vi "Fitter.vi"(8 "error in (no error)":errorcluster, 11 "PmuAnalysis in":refnum<class "FreqAnalysis.lvclass">) -> (0 "error out":errorcluster, 3 "PmuAnalysis out":refnum<class "FreqAnalysis.lvclass">)   [LabVIEW 2018, in "AnalysisPlugins.lvlib" / "FreqAnalysis.lvclass"]
uses:
  FreqAnalysis.lvclass
  C:/projects/ICDAS/NistPluggableModules/Analysis/AnalysisPlugins/AnalysisPluginBaseClass/AnalysisPluginsBase.lvclass
  C:/projects/ICDAS/NistPluggableModules/Analysis/AnalysisPlugins/PmuAnalysisClass/PmuAnalysis.lvclass
  AnalysisPluginBaseClass/AnalysisPluginsBase.lvclass/AnalysisPluginsBase.ctl
  PmuAnalysisClass/Typedefs/PmuData.ctl
  <vilib>/Analysis/coordinate.llb/Angle Units.ctl
  <vilib>/Analysis/coordinate.llb/Angle Range (Degree).ctl
  FitterBaseClass/Typedefs/clAnalysisConfig.ctl
  PmuAnalysisClass/PmuAnalysis.lvclass/PmuAnalysis.ctl
  <vilib>/Analysis/coordinate.llb/Wrap Angle (scalar).vi
  PmuAnalysisClass/Accessors/Read eTestType.vi
  AnalysisPluginBaseClass/Accessors/Read DelayCorr.vi
  AnalysisPluginBaseClass/Accessors/Read MagCorr.vi
  AnalysisPluginBaseClass/Accessors/Read AnalysisConfig.vi
  PmuAnalysisClass/Accessors/Read Function.vi
  PmuAnalysisClass/Accessors/Write Reference.vi
  AnalysisPluginBaseClass/Accessors/Read Window.vi
  <vilib>/Utility/error.llb/Error Cluster From Error Code.vi
  FGen/MemberClasses/FunctionBaseClass/FunctionBase.lvclass
  <vilib>/ErrorRing/Error Ring.xnode
  <vilib>/Analysis/NI_AAL_Angle.lvlib
  PmuAnalysisClass/PmuAnalysis.lvclass
  FitterBaseClass/FitterBase.lvclass
panel:
  out "Phase (rad)":dbl[](array[numeric])
  out "Magnitude":dbl[](array[numeric])
  out "Waveform Graph":dbl[][](graph)
  out "iterations":i32[](array[numeric])
  out "theta":dbl
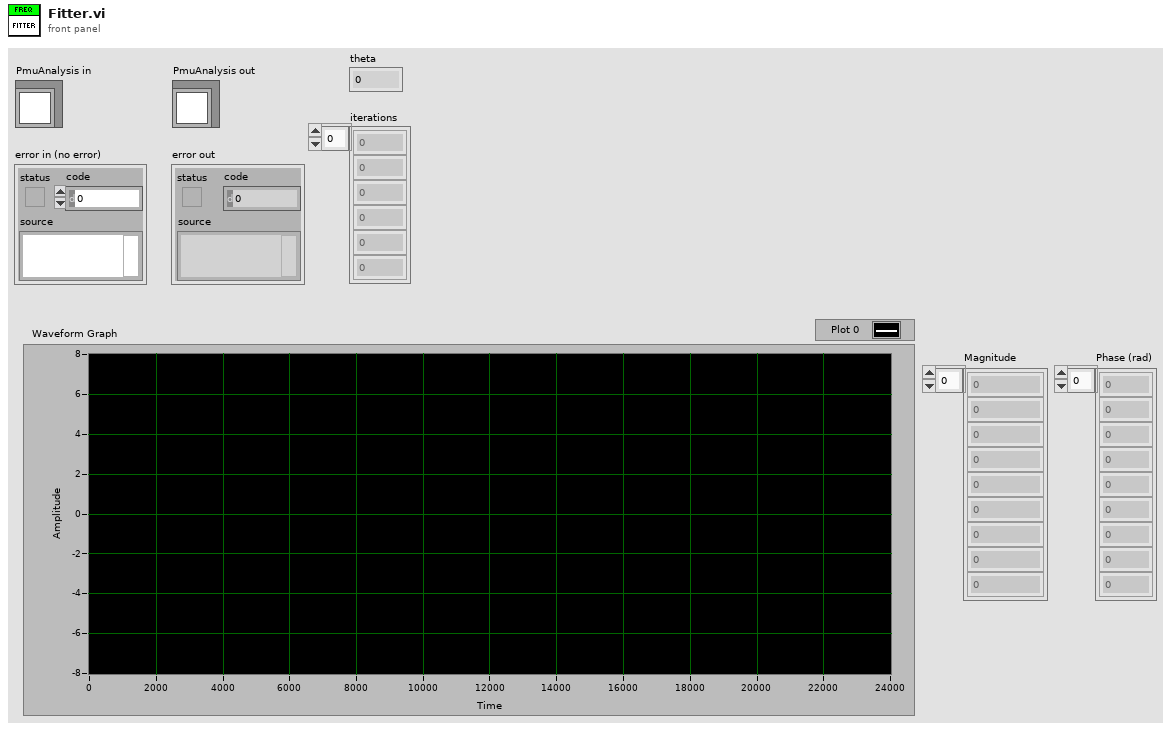
[diagram p1: front panel]
types:
  T1 = typedef "AnalysisPlugins.lvlib/FitterBase.lvclass/clAnalysisConfig.ctl" = cluster{"F0":u32, "SettlingTime":dbl, "AnalysisCycles":dbl, "SampleRate":dbl, "NumChannels":u32, "TsOffset":enum16{"start", "middle", "end"}}
  T2 = typedef "AnalysisPlugins.lvlib/PmuAnalysis.lvclass/PmuData.ctl" = cluster{"Timestamp":dbl, "Synx":cdb[], "Freq":dbl, "ROCOF":dbl, "ID":i16}
  T3 = typedef "AnalysisPlugins.lvlib/AnalysisPluginsBase.lvclass/clWindowData.ctl" = cluster{"Timestamp":ext, "Samples":dbl[][], "Window Valid":bool, "T0":ext}
  T4 = typedef "NI_AAL_Angle.lvlib/Angle Range (Degree).ctl" = u16
  T5 = typedef "NI_AAL_Angle.lvlib/Angle Units.ctl" = i32
  T6 = enum16{"SteadyState", "Modulation", "Ramp", "Step"}
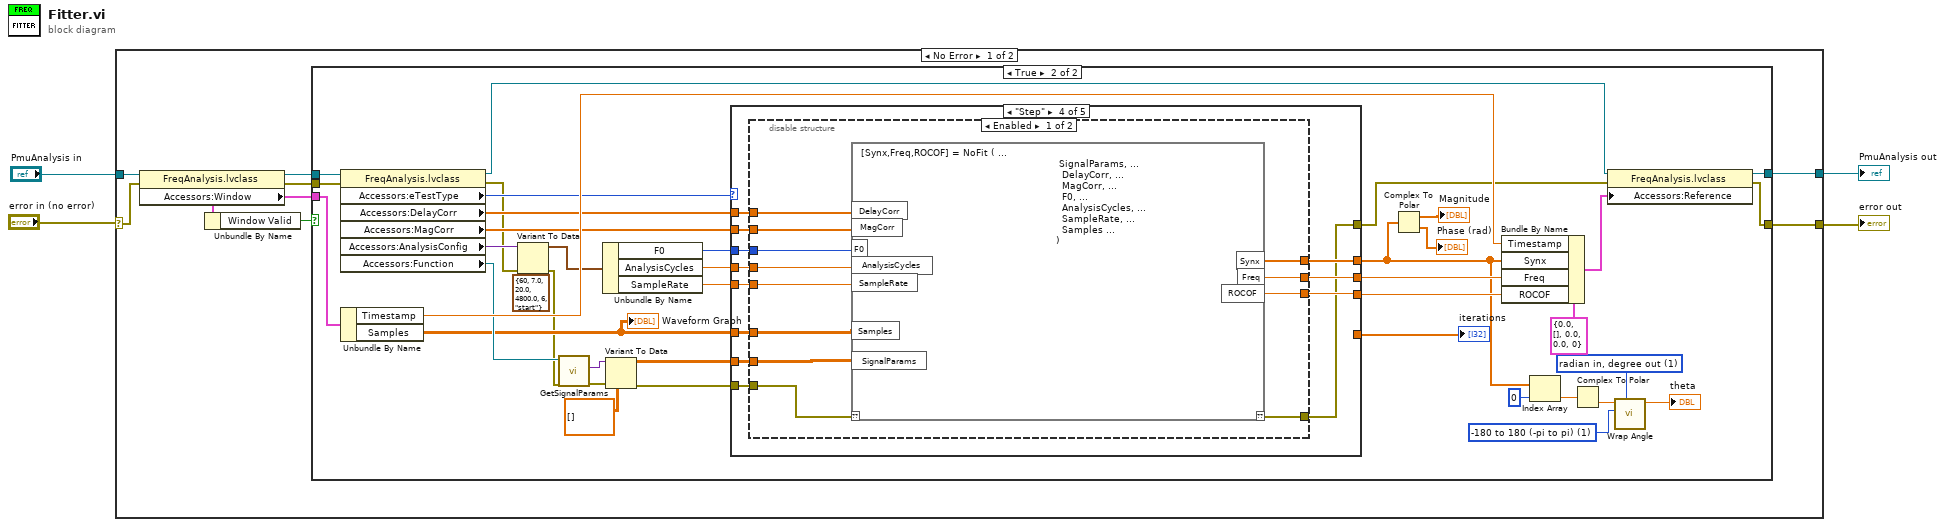
[diagram p0: block diagram]
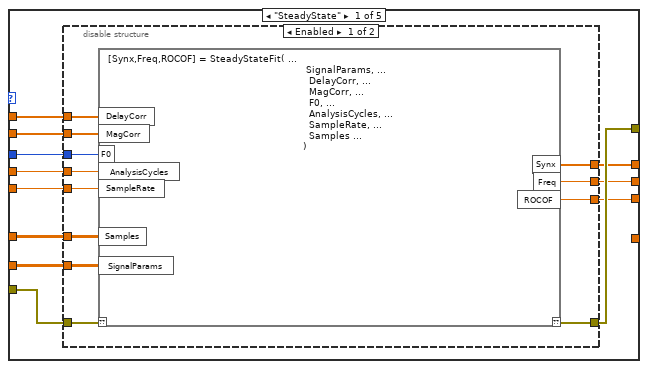
[diagram p3: hidden frame]
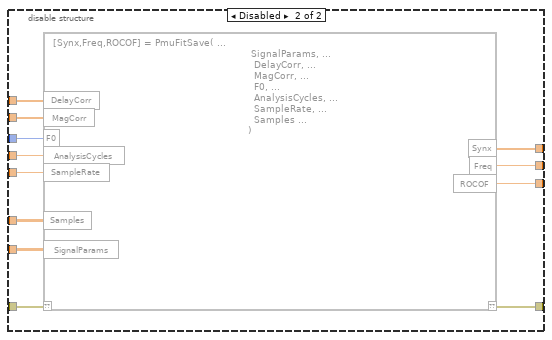
[diagram p4: hidden frame]
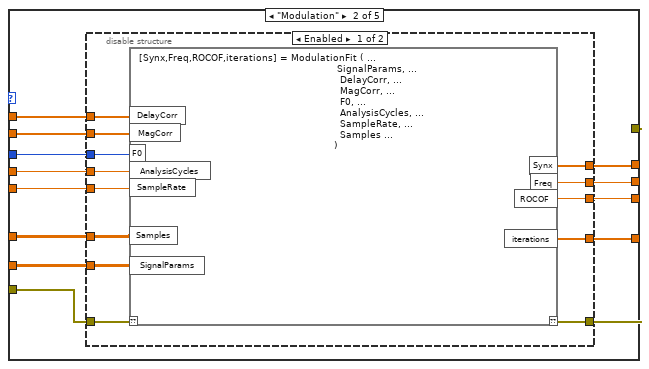
[diagram p5: hidden frame]
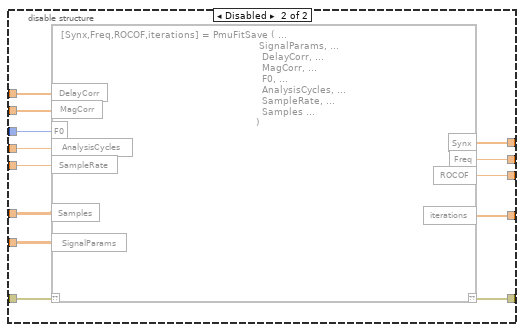
[diagram p6: hidden frame]
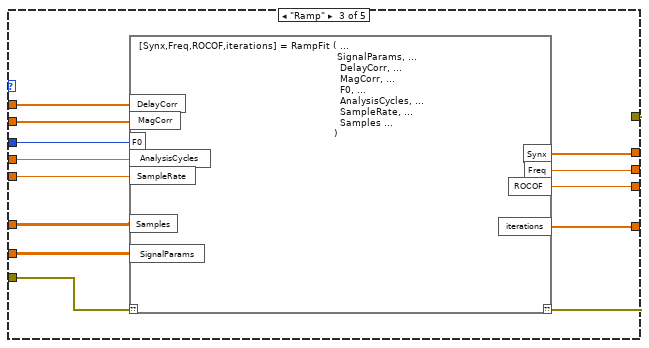
[diagram p7: hidden frame]
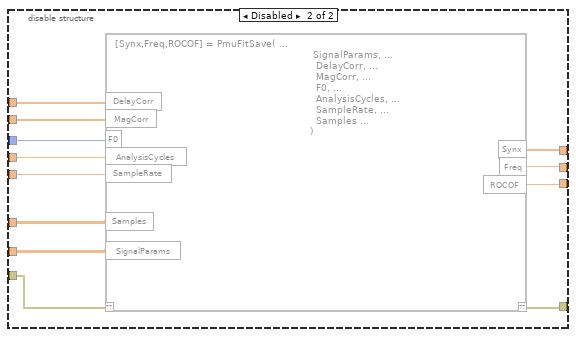
[diagram p8: hidden frame]
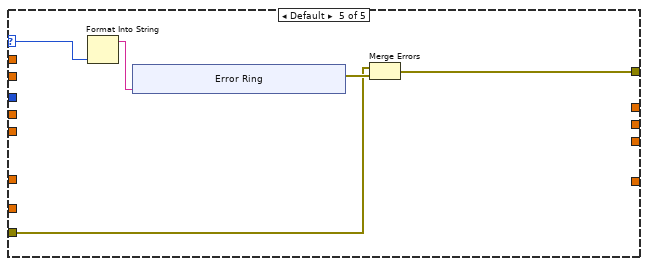
[diagram p9: hidden frame]
diagram:
  n1 = case shown="No Error" "error in (no error)" {
    selector: "error in (no error)" -> [w11 w191]
    tunnel: "PmuAnalysis in" -> [w12 w192]
    tunnel: [w6 w192] -> w2
    tunnel: [w5 w191] -> w1
    frame No Error {
      n2 = property class="FreqAnalysis.lvclass"(reference=w12, error in=w11) -> (reference out=w9:refnum<class "FreqAnalysis.lvclass">, error out=w8:errorcluster, "Accessors:Window"=w7:T3)
      n3 = Unbundle By Name(w7) -> ("Window Valid"=w10:bool)
      n4 = case shown="True" w10 {
        tunnel: w9 -> [w14 w54]
        tunnel: w8 -> [w13 w53]
        tunnel: w7 -> [_ w50]
        tunnel: [w14 w52] -> w6
        tunnel: [w13 w25] -> w5
        frame False {
        }
        frame True {
          w34 = T4 1 items=["none", "-180 to 180 (-pi to pi)", "0 to 360 (0 to 2pi)"] ("angle range")
          w35 = T5 1 items=["radian in, radian out", "radian in, degree out", "degree in, degree out", "degree in, radian out"] ("angle units")
          n5 = property class="FreqAnalysis.lvclass"(reference=w54, error in=w53) -> (reference out=w40:refnum<class "FreqAnalysis.lvclass">, error out=w21:errorcluster, "Accessors:eTestType"=w28:T6, "Accessors:DelayCorr"=w45:dbl[], "Accessors:MagCorr"=w44:dbl[], "Accessors:AnalysisConfig"=w24:variant, "Accessors:Function"=w32:refnum<class "FunctionBase.lvclass">)
          n6 = Unbundle By Name(w50) -> ("Timestamp"=w49:ext, "Samples"=w27:dbl[][])
          "Waveform Graph" <- w27
          n7 = Variant To Data(error in=w21, type=T1 {"F0"=60, "SettlingTime"=7.0, "AnalysisCycles"=20.0, "SampleRate"=4800.0, "NumChannels"=6, "TsOffset"=enum."start"} ("clAnalysisConfig"), Variant=w24) -> (data=w22:T1, error out=w20:errorcluster)
          n8 = call-dynamic "GetSignalParams.vi"("error in (no error)"=w20, "FunctionBase in"=w32) -> ("error out"=w31:errorcluster, "Params"=w30:variant)  [unwired: 7 in, 1 out]
          n9 = Unbundle By Name(w22) -> ("F0"=w43:u32, "AnalysisCycles"=w42:dbl, "SampleRate"=w41:dbl)
          n10 = Variant To Data(error in=w31, type=dbl[][] [], Variant=w30) -> (data=w19:dbl[][], error out=w18:errorcluster)
          n11 = case shown="\"Step\"" w28 {
            selector: w28 -> [_ _ _ _ w181]
            tunnel: [w66 w93 w132 w145 w183] -> w26
            tunnel: w27 -> [w60 w98 w137 w149 _]
            tunnel: [w55 w97 w136 w148 _] -> w15
            tunnel: [w58 w96 w135 w147 _] -> w47
            tunnel: [w59 w95 w134 w146 _] -> w46
            tunnel: w45 -> [w65 w103 w142 w154 _]
            tunnel: w44 -> [w64 w102 w141 w153 _]
            tunnel: w43 -> [w63 w101 w140 w152 _]
            tunnel: w42 -> [w62 w100 w139 w151 _]
            tunnel: w41 -> [w61 w99 w138 w150 _]
            tunnel: [_ w94 w133 _ _] -> w33
            tunnel: w18 -> [w57 w92 w131 w144 w179]
            tunnel: w19 -> [w56 w91 w130 w143 _]
            frame "SteadyState" {
              n12 = disable-structure shown="Enabled" {
                disable-tunnel: [w78 w90] -> w66
                disable-tunnel: w65 -> [w77 w89]
                disable-tunnel: w64 -> [w76 w88]
                disable-tunnel: w63 -> [w75 w87]
                disable-tunnel: w62 -> [w74 w86]
                disable-tunnel: w61 -> [w73 w85]
                disable-tunnel: w60 -> [w72 w84]
                disable-tunnel: [w71 w83] -> w59
                disable-tunnel: [w70 w82] -> w58
                disable-tunnel: w57 -> [w69 w81]
                disable-tunnel: w56 -> [w67 w79]
                disable-tunnel: [w68 w80] -> w55
                frame Enabled {
                  n13 = script code="[Synx,Freq,ROCOF] = SteadyStateFit( ...\n                                                                  SignalParams, ...\n                                                                   DelayCorr, ...\n                                                                   MagCorr, ...\n                                                                   F0, ...\n                                                                   AnalysisCycles, ...\n                                                                   SampleRate, ...\n                                                                   Samples ...\n                                                                 )"("??"=w69, "SignalParams"=w67, "DelayCorr"=w77, "MagCorr"=w76, "F0"=w75, "AnalysisCycles"=w74, "SampleRate"=w73, "Samples"=w72) -> ("??"=w78:errorcluster, "Synx"=w68:cdb[], "Freq"=w70:dbl, "ROCOF"=w71:dbl)
                }
                frame Disabled {
                  n14 = script code="[Synx,Freq,ROCOF] = PmuFitSave( ...\n                                                                  SignalParams, ...\n                                                                   DelayCorr, ...\n                                                                   MagCorr, ...\n                                                                   F0, ...\n                                                                   AnalysisCycles, ...\n                                                                   SampleRate, ...\n                                                                   Samples ...\n                                                                 )"("??"=w81, "SignalParams"=w79, "DelayCorr"=w89, "MagCorr"=w88, "F0"=w87, "AnalysisCycles"=w86, "SampleRate"=w85, "Samples"=w84) -> ("??"=w90:errorcluster, "Synx"=w80:cdb[], "Freq"=w82:dbl, "ROCOF"=w83:dbl)
                }
              }
            }
            frame "Modulation" {
              n15 = disable-structure shown="Enabled" {
                disable-tunnel: w103 -> [w116 w129]
                disable-tunnel: w102 -> [w115 w128]
                disable-tunnel: w101 -> [w114 w127]
                disable-tunnel: w100 -> [w113 w126]
                disable-tunnel: w99 -> [w112 w125]
                disable-tunnel: w98 -> [w111 w124]
                disable-tunnel: [w110 w123] -> w97
                disable-tunnel: [w109 w122] -> w96
                disable-tunnel: [w108 w121] -> w95
                disable-tunnel: [w107 w120] -> w94
                disable-tunnel: [w106 w119] -> w93
                disable-tunnel: w92 -> [w105 w118]
                disable-tunnel: w91 -> [w104 w117]
                frame Enabled {
                  n16 = script code="[Synx,Freq,ROCOF,iterations] = ModulationFit ( ...\n                                                                  SignalParams, ...\n                                                                   DelayCorr, ...\n                                                                   MagCorr, ...\n                                                                   F0, ...\n                                                                   AnalysisCycles, ...\n                                                                   SampleRate, ...\n                                                                   Samples ...\n                                                                 )"("??"=w105, "SignalParams"=w104, "DelayCorr"=w116, "MagCorr"=w115, "F0"=w114, "AnalysisCycles"=w113, "SampleRate"=w112, "Samples"=w111) -> ("??"=w106:errorcluster, "Synx"=w110:cdb[], "Freq"=w109:dbl, "ROCOF"=w108:dbl, "iterations"=w107:dbl[])
                }
                frame Disabled {
                  n17 = script code="[Synx,Freq,ROCOF,iterations] = PmuFitSave ( ...\n                                                                  SignalParams, ...\n                                                                   DelayCorr, ...\n                                                                   MagCorr, ...\n                                                                   F0, ...\n                                                                   AnalysisCycles, ...\n                                                                   SampleRate, ...\n                                                                   Samples ...\n                                                                 )"("??"=w118, "SignalParams"=w117, "DelayCorr"=w129, "MagCorr"=w128, "F0"=w127, "AnalysisCycles"=w126, "SampleRate"=w125, "Samples"=w124) -> ("??"=w119:errorcluster, "Synx"=w123:cdb[], "Freq"=w122:dbl, "ROCOF"=w121:dbl, "iterations"=w120:dbl[])
                }
              }
            }
            frame "Ramp" {
              n18 = script code="[Synx,Freq,ROCOF,iterations] = RampFit ( ...\n                                                                  SignalParams, ...\n                                                                   DelayCorr, ...\n                                                                   MagCorr, ...\n                                                                   F0, ...\n                                                                   AnalysisCycles, ...\n                                                                   SampleRate, ...\n                                                                   Samples ...\n                                                                 )"("??"=w131, "SignalParams"=w130, "DelayCorr"=w142, "MagCorr"=w141, "F0"=w140, "AnalysisCycles"=w139, "SampleRate"=w138, "Samples"=w137) -> ("??"=w132:errorcluster, "Synx"=w136:cdb[], "Freq"=w135:dbl, "ROCOF"=w134:dbl, "iterations"=w133:dbl[])
            }
            frame "Step" {
              n19 = disable-structure shown="Enabled" {
                disable-tunnel: w154 -> [w166 w178]
                disable-tunnel: w153 -> [w165 w177]
                disable-tunnel: w152 -> [w164 w176]
                disable-tunnel: w151 -> [w163 w175]
                disable-tunnel: w150 -> [w162 w174]
                disable-tunnel: w149 -> [w161 w173]
                disable-tunnel: [w160 w167] -> w148
                disable-tunnel: [w159 w168] -> w147
                disable-tunnel: [w158 w169] -> w146
                disable-tunnel: [w157 w170] -> w145
                disable-tunnel: w144 -> [w156 w171]
                disable-tunnel: w143 -> [w155 w172]
                frame Enabled {
                  n20 = script code="[Synx,Freq,ROCOF] = NoFit ( ...\n                                                                  SignalParams, ...\n                                                                   DelayCorr, ...\n                                                                   MagCorr, ...\n                                                                   F0, ...\n                                                                   AnalysisCycles, ...\n                                                                   SampleRate, ...\n                                                                   Samples ...\n                                                                 )"("??"=w156, "SignalParams"=w155, "DelayCorr"=w166, "MagCorr"=w165, "F0"=w164, "AnalysisCycles"=w163, "SampleRate"=w162, "Samples"=w161) -> ("??"=w157:errorcluster, "Synx"=w160:cdb[], "Freq"=w159:dbl, "ROCOF"=w158:dbl)
                }
                frame Disabled {
                  n21 = script code="[Synx,Freq,ROCOF] = PmuFitSave( ...\n                                                                  SignalParams, ...\n                                                                   DelayCorr, ...\n                                                                   MagCorr, ...\n                                                                   F0, ...\n                                                                   AnalysisCycles, ...\n                                                                   SampleRate, ...\n                                                                   Samples ...\n                                                                 )"("??"=w171, "SignalParams"=w172, "DelayCorr"=w178, "MagCorr"=w177, "F0"=w176, "AnalysisCycles"=w175, "SampleRate"=w174, "Samples"=w173) -> ("??"=w170:errorcluster, "Synx"=w167:cdb[], "Freq"=w168:dbl, "ROCOF"=w169:dbl)
                }
              }
            }
            frame Default {
              n22 = Format Into String(w181) -> (resulting string=w180:string)  [unwired: 3 in, 1 out]
              n23 = xnode "Error Ring"("parameter 0"=w180) -> ("error out"=w182:errorcluster)
              n24 = Merge Errors(w179, w182) -> (w183:errorcluster)
            }
          }
          "iterations" <- w33
          n25 = Complex To Polar(r * e^(i*theta)=w15) -> (r=→"Magnitude":dbl[], theta=→"Phase (rad)":dbl[])
          n26 = Bundle By Name(cluster=T2 {"Timestamp"=0.0, "Synx"=[], "Freq"=0.0, "ROCOF"=0.0, "ID"=0} ("PmuReport"), "Timestamp"=w49, "Synx"=w15, "Freq"=w47, "ROCOF"=w46) -> (w48:T2)
          n27 = Index Array(array=w15, index=0) -> (element=w38:cdb)
          n28 = Complex To Polar(r * e^(i*theta)=w38) -> (theta=w37:dbl)  [unwired: 1 out]
          n29 = property class="FreqAnalysis.lvclass"(reference=w40, error in=w26, "Accessors:Reference"=w48) -> (reference out=w52:refnum<class "FreqAnalysis.lvclass">, error out=w25:errorcluster)
          n30 = call-poly <vilib>:"Wrap Angle.vi"("angle units"=w35, "angle range"=w34, "angle in"=w37) -> ("angle out"=→"theta":dbl)  [unwired: 7 in, 1 out]
        }
      }
    }
    frame Error {
    }
  }
  "error out" <- w1
  "PmuAnalysis out" <- w2
